vi "XMLtoGV.vi"() -> ()   [LabVIEW 2014]
uses:
  GV.vi
panel:
  in  "String":string="<xml><name>test</name></xml>"
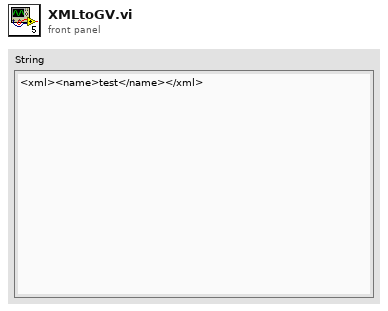
[diagram p1: front panel]
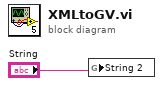
[diagram p0: block diagram]
diagram:
  n1 = global write "GV.vi" "String 2"("String") -> ()
